vi "Close Pop-Up (Two Button Choice).vi"(8 "error in":errorcluster, 10 "Two-Button Choice? (F)":bool) -> (0 "error out":errorcluster)   [LabVIEW 2021, in "Pop-Up.lvlib" / "Popup.lvclass"]
doc: "This VI can be used to close the pop-up early before the user has finished interacting.\n\nUse this VI to also send a Boolean value - this is read when using the two-button dialog pop-up types (timeout or standard). This will make the selection for the user based on whatever the developer has decided. \n\n<b>Code Developed By:</b>\nTechnology Service Corporation\n1983 S Liberty Drive\nBloomington, IN 47403\nPhone: 812 558-7100\nwww.tsc.com/atcs\n\nDeveloper:\nDaniel Coons"
uses:
  Popup.lvclass
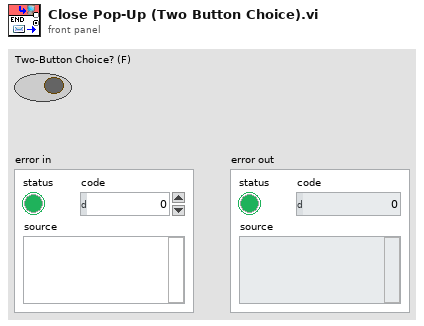
[diagram p1: front panel]
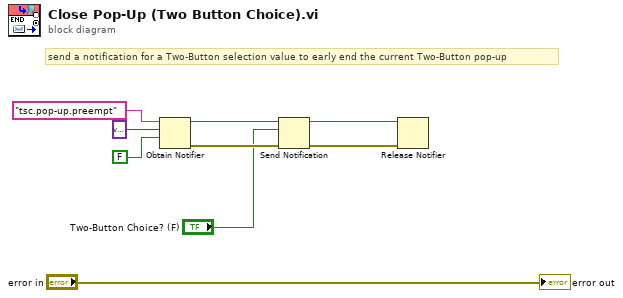
[diagram p0: block diagram]
diagram:
  # "send a notification for a Two-Button selection value to early end the current Two-Button pop-up"
  n1 = Obtain Notifier(name (unnamed)="tsc.pop-up.preempt", notification data type=variant, create if not found? (T)=FALSE) -> (notifier out=w4:refnum<notifier>, error out=w6:errorcluster)  [unwired: 1 in, 1 out]
  n2 = Send Notification(notification="Two-Button Choice? (F)", notifier=w4, error in (no error)=w6) -> (notifier out=w3:refnum<notifier>, error out=w5:errorcluster)
  n3 = Release Notifier(notifier=w3, error in (no error)=w5) -> ()  [unwired: 1 in, 3 out]
  "error out" <- "error in"
